vi "spi_raw.vi"() -> ()   [LabVIEW 2011]
panel:
  out "arrayout 2":u8[](array[numeric]) format="%.0x"
  out "Error":errorcluster caption="error"
  out "arrayout":u8[](array[numeric]) format="%.0x"
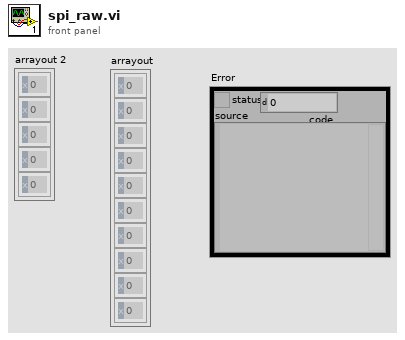
[diagram p1: front panel]
types:
  T1 = typedef "IOWarrior_Handle.ctl" = cluster{"Handle":u32, "Serial Number":string, "type of Warrior":T2, "Root Handle":bool, "Revision":u16}
  T2 = typedef "IOWarrior_Type.ctl" = enum16{"invalid", "IOW24", "IOW40", "IOW56", "IOPV1", "IOPV2"}
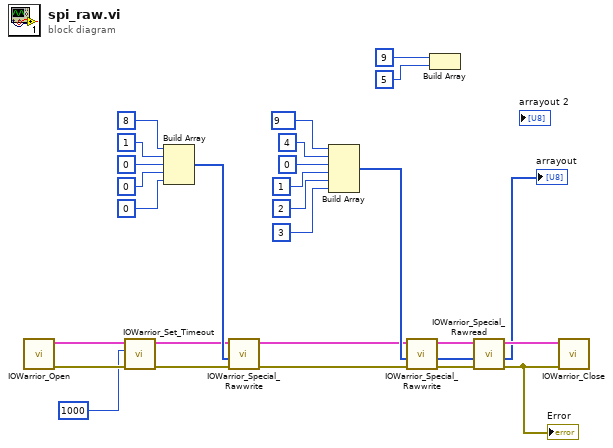
[diagram p0: block diagram]
diagram:
  n1 = call "IOWarrior_Open.vi"() -> ("err out"=w3:errorcluster, "IOWarriorHandle"=w6:T1)  [unwired: 9 in, 1 out]
  n2 = call "IOWarrior_Set_Timeout.vi"("err in"=w3, "timeout_ms(1000)"=1000, "devHandle"=w6) -> ("err out"=w4:errorcluster, "devHandleout"=w5:T1)  [unwired: 6 in, 1 out]
  n3 = Build Array(u8 8, u8 1, u8 0, u8 0, u8 0) -> (w23:u8[])
  n4 = call "IOWarrior_Special_Rawwrite.vi"("err in"=w4, "Array_in"=w23, "devHandle"=w5) -> ("err out"=w15:errorcluster, "devHandleout"=w16:T1)  [unwired: 6 in, 1 out]
  n5 = Build Array(u8 9, u8 4, u8 0, u8 1, u8 2, u8 3) -> (w17:u8[])
  n6 = call "IOWarrior_Special_Rawwrite.vi"("err in"=w15, "Array_in"=w17, "devHandle"=w16) -> ("err out"=w13:errorcluster, "array_out"=w1:u8[], "devHandleout"=w14:T1)  [unwired: 6 in]
  n7 = Build Array(u8 9, u8 5) -> ()  [unwired: 1 out]
  n8 = call "IOWarrior_Special_Rawread.vi"("err in"=w13, "array"=w1, "devHandle"=w14) -> ("err out"=w9:errorcluster, "arrayout"=→"arrayout":u8[], "devHandleout"=w12:T1)  [unwired: 6 in]
  "Error" <- w9
  n9 = call "IOWarrior_Close.vi"("err in"=w9, "devHandle"=w12) -> ()  [unwired: 8 in, 2 out]
